vi "Test Program.vi"() -> ()   [LabVIEW 2018]
doc: "Test Program.vi\n\nThis is a simple program that uses the ICM to demonstrate its structure.\n\nInstrument Communication Module Version 1.0\nDecember, 2017 Original Code Consulting David Thomson\n www.originalcode.com"
uses:
  Scaling/Scaling.lvclass
  Scaling/Scaling.lvclass/Scaling.ctl
  Query/Query.lvclass/Query.ctl
  Query/Read Cycle Time (ms).vi
  Initialize/Initialize.lvclass
  Parser/Parser.lvclass
  Output/Output.lvclass
  Query/Query.lvclass
  Bus/Bus.lvclass
panel:
  in  "Controller Values":dbl[](array[numeric])
  out "Enabled Controllers":string[](array[string])
  out "Scaled Values":dbl[](array[numeric])
  in  "stop":bool
  out "Enabled Channels":string[](array[string])
  out "Data Values":dbl[](array[numeric])
  out "String Read":string
  out "error out":errorcluster
  out "Config File":path
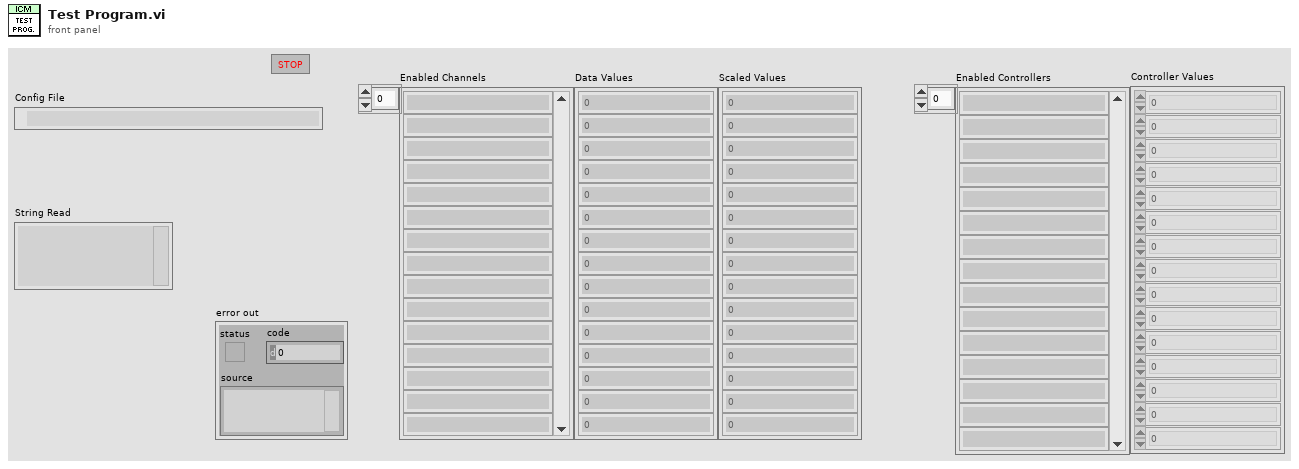
[diagram p1: front panel]
types:
  T1 = typedef "Scaling Def.ctl" = cluster{"Channel":string, "Scaling":string, "Instance":string}
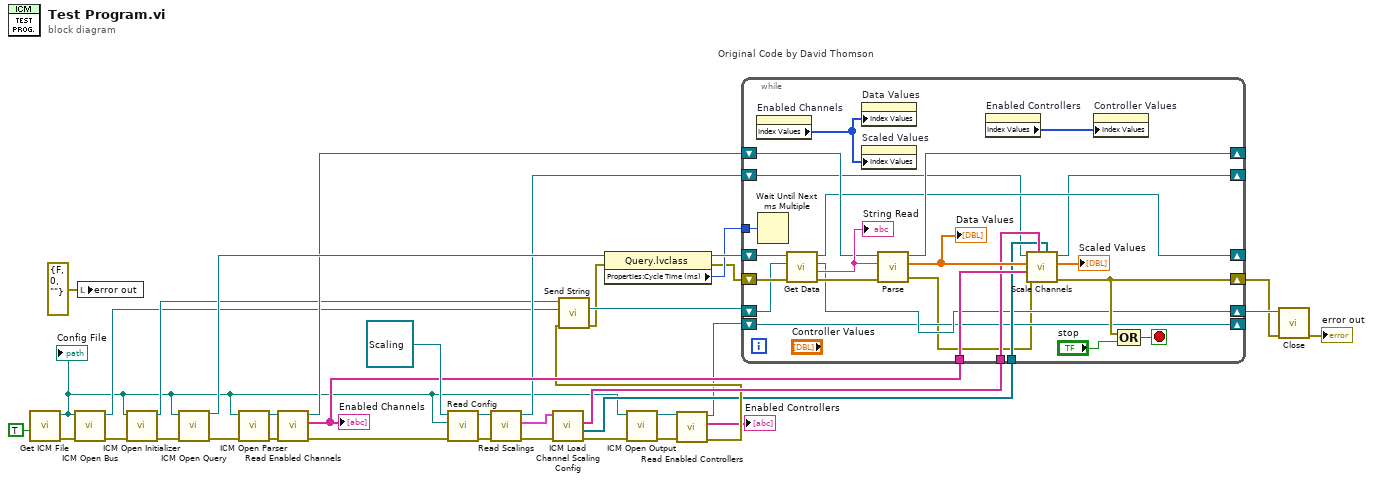
[diagram p0: block diagram]
diagram:
  n1 = call "Get ICM File.vi"("Re-Init?"=TRUE) -> ("error out"=w30:errorcluster, "ICM File"=w5:path)  [unwired: 9 in]
  "Config File" <- w5
  n2 = call "ICM Open Bus.vi"("error in (no error)"=w30, "ICM File In"=w5) -> ("error out"=w14:errorcluster, "Bus out"=w12:refnum<class "Bus.lvclass">)  [unwired: 8 in]
  n3 = local write "error out"(errorcluster {"status"=FALSE, "code"=0, "source"=""} ("error out")) -> ()
  n4 = call "ICM Open Initializer.vi"("error in (no error)"=w14, "ICM File In"=w5) -> ("error out"=w1:errorcluster, "Init out"=w13:refnum<class "Initialize.lvclass">)  [unwired: 8 in]
  n5 = call "ICM Open Query.vi"("error in (no error)"=w1, "ICM File In"=w5) -> ("error out"=w31:errorcluster, "Query out"=w21:refnum<class "Query.lvclass">)  [unwired: 8 in]
  n6 = call "ICM Open Parser.vi"("error in (no error)"=w31, "ICM File In"=w5) -> ("error out"=w32:errorcluster, "Parser out"=w33:refnum<class "Parser.lvclass">)  [unwired: 8 in]
  n7 = call-dynamic "Read Enabled Channels.vi"("error in (no error)"=w32, "Parser in"=w33) -> ("error out"=w29:errorcluster, "Enabled Channels"=w27:string[], "Parser out"=w16:refnum<class "Parser.lvclass">)  [unwired: 7 in]
  "Enabled Channels" <- w27
  n8 = call-dynamic "Read Config.vi"("error in (no error)"=w29, "ICM File In"=w5, "Scaling in"=refnum<class "Scaling.lvclass"> refnum) -> ("error out"=w25:errorcluster, "Scaling out"=w23:refnum<class "Scaling.lvclass">)  [unwired: 7 in]
  n9 = call "Read Scalings.vi"("error in (no error)"=w25, "Scaling in"=w23) -> ("error out"=w24:errorcluster, "Scalings"=w22:T1[], "Scaling out"=w15:refnum<class "Scaling.lvclass">)  [unwired: 7 in]
  n10 = call "ICM Load Channel Scaling Config.vi"("error in (no error)"=w24, "Scalings"=w22) -> ("error out"=w7:errorcluster, "Scaling Classes"=w8:refnum<class "Scaling.lvclass">[], "Used Scalings"=w26:string[])  [unwired: 6 in, 1 out]
  n11 = call "ICM Open Output.vi"("error in (no error)"=w7, "ICM File In"=w5) -> ("error out"=w6:errorcluster, "Output out"=w4:refnum<class "Output.lvclass">)  [unwired: 8 in]
  n12 = call-dynamic "Read Enabled Controllers.vi"("error in (no error)"=w6, "Output in"=w4) -> ("error out"=w9:errorcluster, "Enabled Channels"=→"Enabled Controllers":string[], "Output out"=w2:refnum<class "Output.lvclass">)  [unwired: 7 in]
  n13 = call-dynamic "Send String.vi"("error in (no error)"=w9, "Bus In"=w12, "Init in"=w13) -> ("error out"=w10:errorcluster, "Bus Out"=w11:refnum<class "Bus.lvclass">)  [unwired: 4 in, 1 out]
  n14 = property class="Query.lvclass"(reference=w21, error in=w10) -> (reference out=w20:refnum<class "Query.lvclass">, error out=w18:errorcluster, "Properties:Cycle Time (ms)"=w19:u32)
  n15 = while "Original Code by David Thomson" {
    shift-right: [w53] -> w35
    shift-left: w18 -> [w59]
    tunnel: w19 -> [w55]
    tunnel: w27 -> [w51]
    tunnel: w26 -> [w49]
    tunnel: w8 -> [w48]
    shift-right: [w42] -> w36
    shift-left: w11 -> [w54]
    shift-right: [w46] -> _
    shift-left: w16 -> [w47]
    shift-right: [w45] -> _
    shift-left: w20 -> [w60]
    shift-right: [w43] -> _
    shift-left: w15 -> [w44]
    shift-right: [w41] -> _
    shift-left: w2 -> [w41]
    stop <- w57 stop-if-true
    n16 = property on="Enabled Channels" class="Arr (strict)"() -> ("Index Values"=w39:u32[])  [unwired: 2 in, 2 out]
    n17 = Wait Until Next ms Multiple(millisecond multiple=w55) -> ()  [unwired: 1 out]
    n18 = call-dynamic "Get Data.vi"("error in (no error)"=w59, "Bus In"=w54, "Query in"=w60) -> ("error out"=w58:errorcluster, "String Read"=w61:string, "Bus Out"=w42:refnum<class "Bus.lvclass">, "Query out"=w45:refnum<class "Query.lvclass">)  [unwired: 5 in]
    "String Read" <- w61
    n19 = property on="Data Values" class="Arr (strict)"("Index Values"=w39) -> ()  [unwired: 2 in, 2 out]
    n20 = property on="Scaled Values" class="Arr (strict)"("Index Values"=w39) -> ()  [unwired: 2 in, 2 out]
    n21 = call-dynamic "Parse.vi"("error in (no error)"=w58, "Data String"=w61, "Parser in"=w47) -> ("error out"=w40:errorcluster, "Data Values"=w52:dbl[], "Parser out"=w46:refnum<class "Parser.lvclass">)  [unwired: 6 in]
    "Data Values" <- w52
    n22 = property on="Enabled Controllers" class="Arr (strict)"() -> ("Index Values"=w38:u32[])  [unwired: 2 in, 2 out]
    n23 = call "Scale Channels.vi"("Scaling Classes"=w48, "Used Scalings"=w49, "error in (no error)"=w40, "Channel Names"=w51, "Values In"=w52, "Scaling in"=w44) -> ("error out"=w53:errorcluster, "Values Out"=→"Scaled Values":dbl[], "Scaling out"=w43:refnum<class "Scaling.lvclass">)  [unwired: 3 in]
    n24 = property on="Controller Values" class="Arr (strict)"("Index Values"=w38) -> ()  [unwired: 2 in, 2 out]
    n25 = Compound Arithmetic op=OR(w53, "stop") -> (w57:bool)
  }
  n26 = call-dynamic "Close.vi"("error in (no error)"=w35, "Bus in"=w36) -> ("error out"=→"error out":errorcluster)  [unwired: 8 in, 1 out]
